vi "Scripting_AlignToConenctorPane.vi"(8 "error in":errorcluster, 11 "ViRef In":refnum<vi>) -> (0 "error out":errorcluster, 3 "VIRefOut":refnum<vi>)   [LabVIEW 2020, in "Scripting.lvclass"]
uses:
  Scripting.lvclass
  Scripting.lvclass/Scripting.ctl
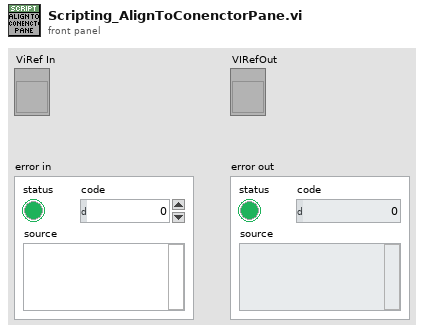
[diagram p1: front panel]
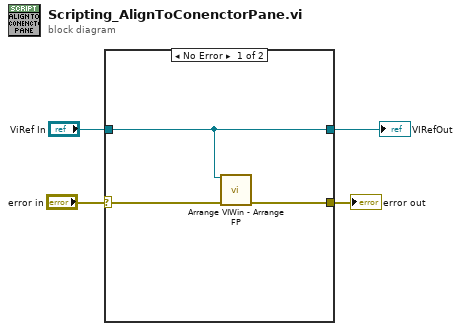
[diagram p0: block diagram]
diagram:
  n1 = case shown="No Error" "error in" {
    selector: "error in" -> [w7 w9]
    tunnel: [w6 w9] -> w3
    tunnel: "ViRef In" -> [w5 w8]
    tunnel: [w5 w8] -> w1
    frame No Error {
      n2 = call <resource>:"Arrange VIWin - Arrange FP.vi"("VI"=w5, "error in"=w7) -> ("error out"=w6:errorcluster)  [unwired: 13 in]
    }
    frame Error {
    }
  }
  "VIRefOut" <- w1
  "error out" <- w3
